vi "Scale Waveform.vi"(8 "Error":errorcluster, 9 "Waveform":T1, 11 "WavBuf":refnum<class "WavBuf.lvclass">) -> (0 "Error Out":errorcluster, 1 "Waveform Out":T1, 3 "WavBuf Out":refnum<class "WavBuf.lvclass">)   [LabVIEW 2025, in "WavBuf.lvclass"]
uses:
  WavBuf.lvclass
  Universal Controls/Waveform_Data.ctl
  WavBuf.lvclass/WavBuf.ctl
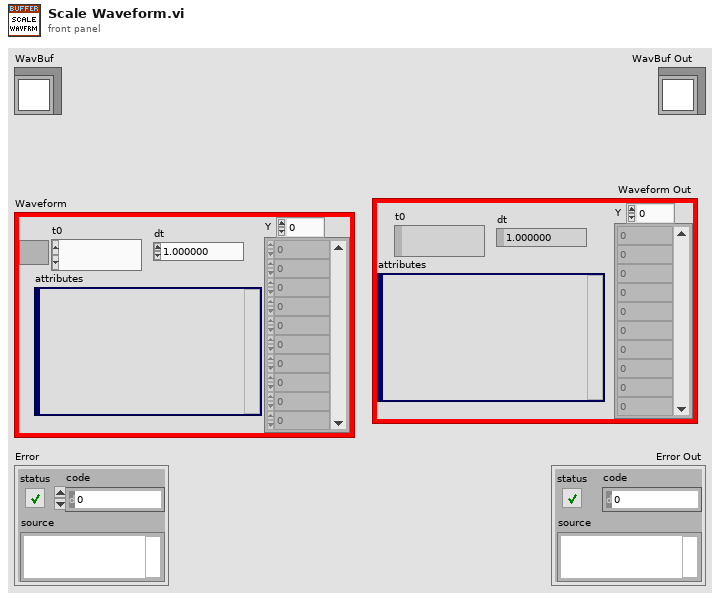
[diagram p1: front panel]
types:
  T1 = typedef "Waveform_Data.ctl" = waveform(dbl)
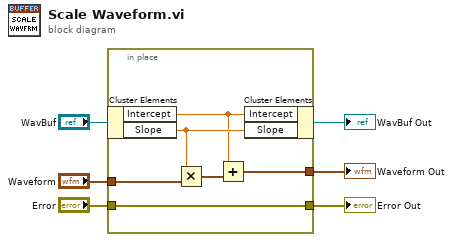
[diagram p0: block diagram]
diagram:
  n1 = in-place {
    in-place-border: [w10] -> w6
    in-place-border: [w8] -> w5
    in-place-border: "Waveform" -> [w7]
    in-place-border: "Error" -> [w8]
    n2 = in-place-cluster #1("WavBuf") -> ("Intercept"=w9:dbl, "Slope"=w12:dbl)
    n3 = Multiply(x=w12, y=w7) -> (x*y=w11:T1)
    n4 = Add(x=w9, y=w11) -> (x+y=w10:T1)
    n5 = in-place-cluster #1("Intercept"=w9, "Slope"=w12) -> (→"WavBuf Out":refnum<class "WavBuf.lvclass">)
  }
  "Waveform Out" <- w6
  "Error Out" <- w5
